vi "Calculate Potting Data.vi"(8 "error in":errorcluster, 11 "Potting Procedure in":refnum<class "Potting Procedure.lvclass">) -> (0 "error out":errorcluster, 2 "Module Potting Data":T1[](array[typedef]), 3 "Potting Procedure out":refnum<class "Potting Procedure.lvclass">)   [LabVIEW 2011, in "Potting Procedure.lvclass"]
uses:
  Potting Procedure.lvclass
  Shared Components/SyringeTool Class/Type Definitions/Module Potting Data.ctl
  Shared Components/Utils/Type Definitions/3d Line.ctl
  Shared Components/Vec3d Class/Vec3d Class.lvclass
  Potting Procedure.lvclass/Potting Procedure.ctl
  Shared Components/Gantry Class/Gantry Class.lvclass
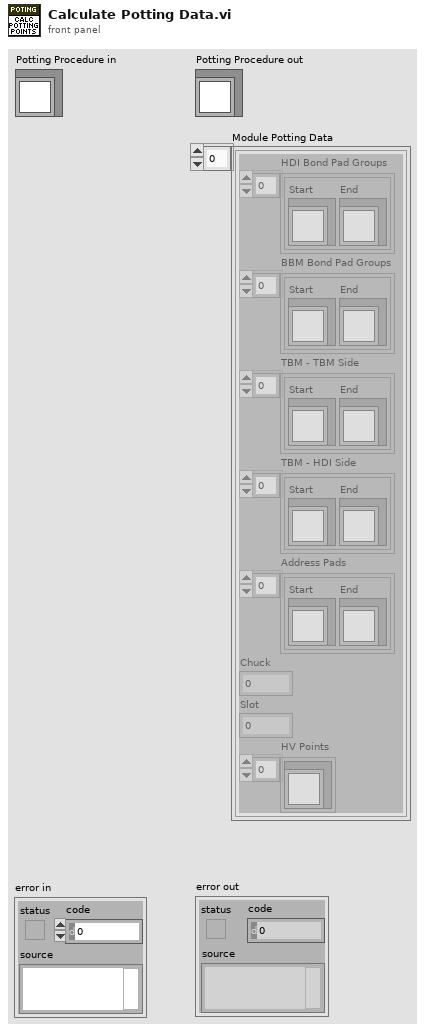
[diagram p1: front panel]
types:
  T1 = typedef "Module Potting Data.ctl" = cluster{"HDI Bond Pad Groups":T2[], "BBM Bond Pad Groups":T2[], "TBM - TBM Side":T2[], "TBM - HDI Side":T2[], "Address Pads":T2[], "Chuck":i32, "Slot":i32, "HV Points":refnum<class "Vec3d Class.lvclass">[]}
  T2 = typedef "3d Line.ctl" = cluster{"Start":refnum<class "Vec3d Class.lvclass">, "End":refnum<class "Vec3d Class.lvclass">}
  T3 = typedef "Inspect Modules - Module.ctl" = cluster{"TBM-TBM":T4, "TBM-HDI":T4, "Address Pads":T4, "HDI Bond Pad References":T8[], "BBM Bond Pad References":T8[], "HV-HDI":T8, "HV-BBM":T8, "Chuck":i32, "Slot":i32, "Potting Selection":cluster{"HDI Bond Pads":bool[], "BBM Bond Pads":bool[], "TBM Inner":cluster{"Top":bool, "Left":bool, "Bottom":bool, "Right":bool}, "TBM Outer":cluster{"Top":bool, "Left":bool, "Bottom":bool, "Right":bool}, "Address Pads":cluster{"Top":bool, "Bottom":bool}, "High Voltage":cluster{"HDI":bool, "Sensor":bool}}}
  T4 = typedef "Multi-Fiducial Image.ctl" = cluster{"Fiducial Image":T5, "Fiducials":cluster{"Selected Fiducial":T7, "fiducial name":string}[]}
  T5 = typedef "Physical Image.ctl" = cluster{"Image Position":refnum<class "Vec3d Class.lvclass">, "Image Reference":T6, "Field of View":cluster{"x(mm)":dbl, "y(mm)":dbl}}
  T6 = typedef "IMAQ Image.ctl" = refnum<image>
  T7 = typedef "Fiducial with Source.ctl" = cluster{"Fiducial Image Coordinate":refnum<class "Vec3d Class.lvclass">, "Fiducial Source":enum16{"Pattern Recognition", "User", "Error", "Default"}}
  T8 = typedef "Fiducial Image.ctl" = cluster{"Fiducial Image":T5, "Selected Fiducial":T7, "fiducial name":string}
  T9 = cluster{"Top":bool, "Left":bool, "Bottom":bool, "Right":bool}
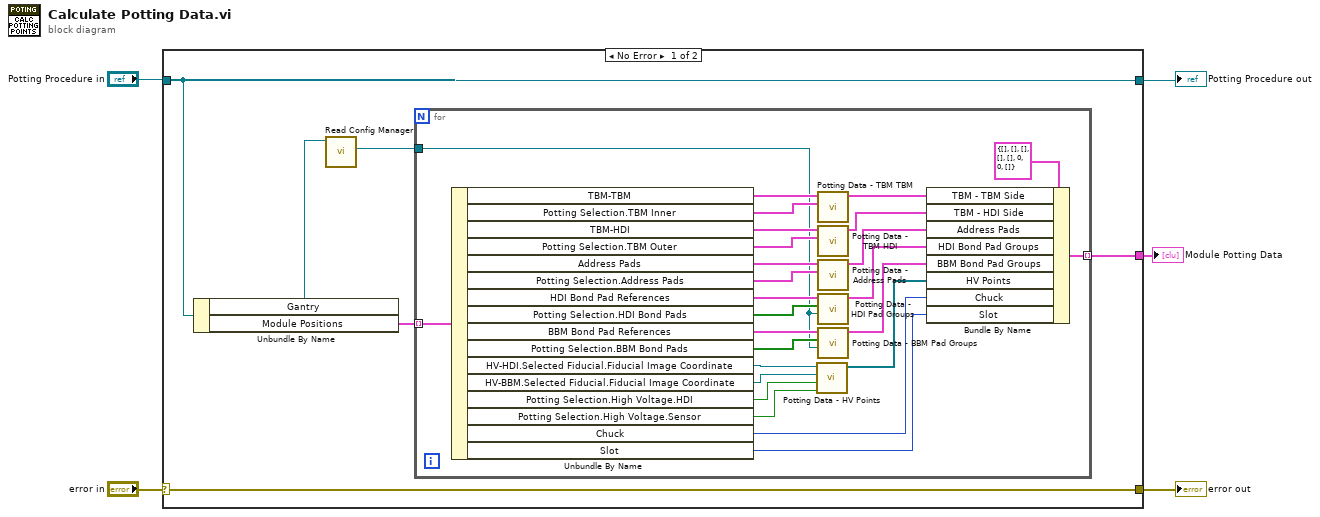
[diagram p0: block diagram]
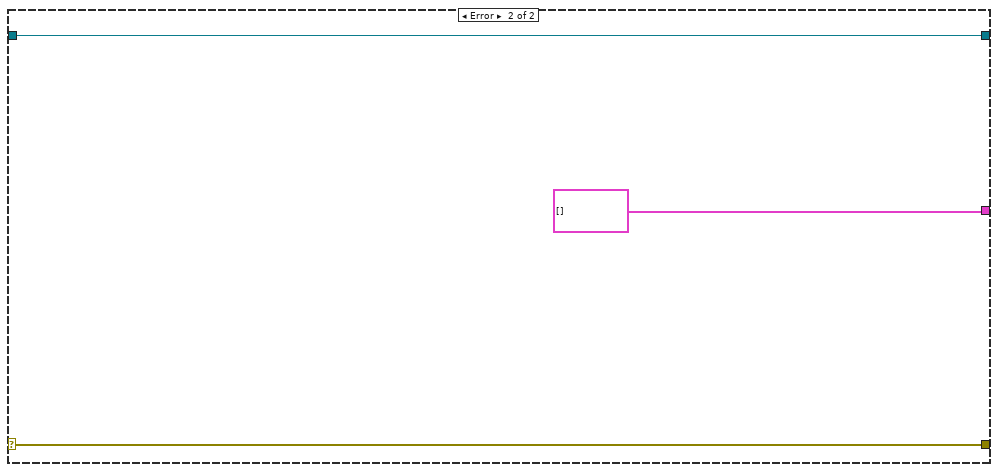
[diagram p2: hidden frame]
diagram:
  n1 = case shown="No Error" "error in" {
    selector: "error in" -> [w11 w40]
    tunnel: [w11 w40] -> w3
    tunnel: "Potting Procedure in" -> [w7 w39]
    tunnel: [w7 w39] -> w2
    tunnel: [w6 T1[] []] -> w1
    frame No Error {
      n2 = Unbundle By Name(w7) -> ("Gantry"=w9:refnum<class "Gantry Class.lvclass">, "Module Positions"=w10:T3[])
      n3 = call-dynamic "Read Config Manager.vi"("Gantry in"=w9) -> ("Config Manager"=w8:refnum<class "Config Manager Class.lvclass">)  [unwired: 8 in, 2 out]
      n4 = for {
        tunnel: w10 -> [w32] mode=indexing
        tunnel: w8 -> [w26]
        tunnel: [w12] -> w6 mode=indexing
        n5 = Unbundle By Name(w32) -> ("TBM-TBM"=w37:T4, "Potting Selection.TBM Inner"=w36:T9, "TBM-HDI"=w35:T4, "Potting Selection.TBM Outer"=w34:T9, "Address Pads"=w31:T4, "Potting Selection.Address Pads"=w33:cluster{"Top":bool, "Bottom":bool}, "HDI Bond Pad References"=w30:T8[], "Potting Selection.HDI Bond Pads"=w29:bool[], "BBM Bond Pad References"=w28:T8[], "Potting Selection.BBM Bond Pads"=w27:bool[], "HV-HDI.Selected Fiducial.Fiducial Image Coordinate"=w17:refnum<class "Vec3d Class.lvclass">, "HV-BBM.Selected Fiducial.Fiducial Image Coordinate"=w16:refnum<class "Vec3d Class.lvclass">, "Potting Selection.High Voltage.HDI"=w15:bool, "Potting Selection.High Voltage.Sensor"=w14:bool, "Chuck"=w24:i32, "Slot"=w23:i32)
        n6 = call "Potting Data - HV Points.vi"("Selection Sensor"=w14, "Selection HDI"=w15, "HV-Sensor"=w16, "HV-HDI"=w17) -> ("HV Potting Points"=w13:refnum<class "Vec3d Class.lvclass">[])  [unwired: 7 in]
        n7 = call "Potting Data - TBM TBM.vi"("TBM-TBM Selection"=w36, "TBM-TBM Data"=w37) -> ("Potting Lines"=w22:T2[])  [unwired: 9 in]
        n8 = call "Potting Data - TBM HDI.vi"("TBM-HDI Selection"=w34, "TBM-HDI Data"=w35) -> ("Potting Lines"=w21:T2[])  [unwired: 9 in]
        n9 = call "Potting Data - Address Pads.vi"("Address Pads Selection"=w33, "Address Pads Data"=w31) -> ("Potting Lines"=w20:T2[])  [unwired: 9 in]
        n10 = call "Potting Data - HDI Pad Groups.vi"("Config Manager"=w26, "Potting Selection HDI Bond Pads"=w29, "HDI Bond Pad References"=w30) -> ("Potting Lines"=w19:T2[])  [unwired: 7 in, 1 out]
        n11 = call "Potting Data - BBM Pad Groups.vi"("Config Manager"=w26, "Potting Selection BBM Bond Pads"=w27, "BBM Bond Pad References"=w28) -> ("Potting Lines"=w18:T2[])  [unwired: 7 in, 1 out]
        n12 = Bundle By Name(cluster=T1 {"HDI Bond Pad Groups"=[], "BBM Bond Pad Groups"=[], "TBM - TBM Side"=[], "TBM - HDI Side"=[], "Address Pads"=[], "Chuck"=0, "Slot"=0, "HV Points"=[]} ("Module Potting Data"), "TBM - TBM Side"=w22, "TBM - HDI Side"=w21, "Address Pads"=w20, "HDI Bond Pad Groups"=w19, "BBM Bond Pad Groups"=w18, "HV Points"=w13, "Chuck"=w24, "Slot"=w23) -> (w12:T1)
      }
    }
    frame Error {
    }
  }
  "error out" <- w3
  "Potting Procedure out" <- w2
  "Module Potting Data" <- w1
